vi "ListBox Auto Resize.vi"(8 "error in (no error)":errorcluster, 9 "Number of Columns":i32=4, 10 "Owning Pane":refnum<vi>, 11 "MultiColumn Listbox":refnum<vi>) -> (0 "error out":errorcluster)   [LabVIEW 2023]
uses:
  <vilib>/Utility/miscctls.llb/LVRowAndColumnTypeDef.ctl
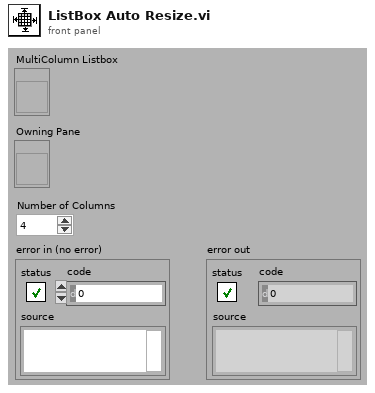
[diagram p1: front panel]
types:
  T1 = typedef "LVRowAndColumnTypeDef.ctl" = cluster{"Row":i32, "Column":i32}
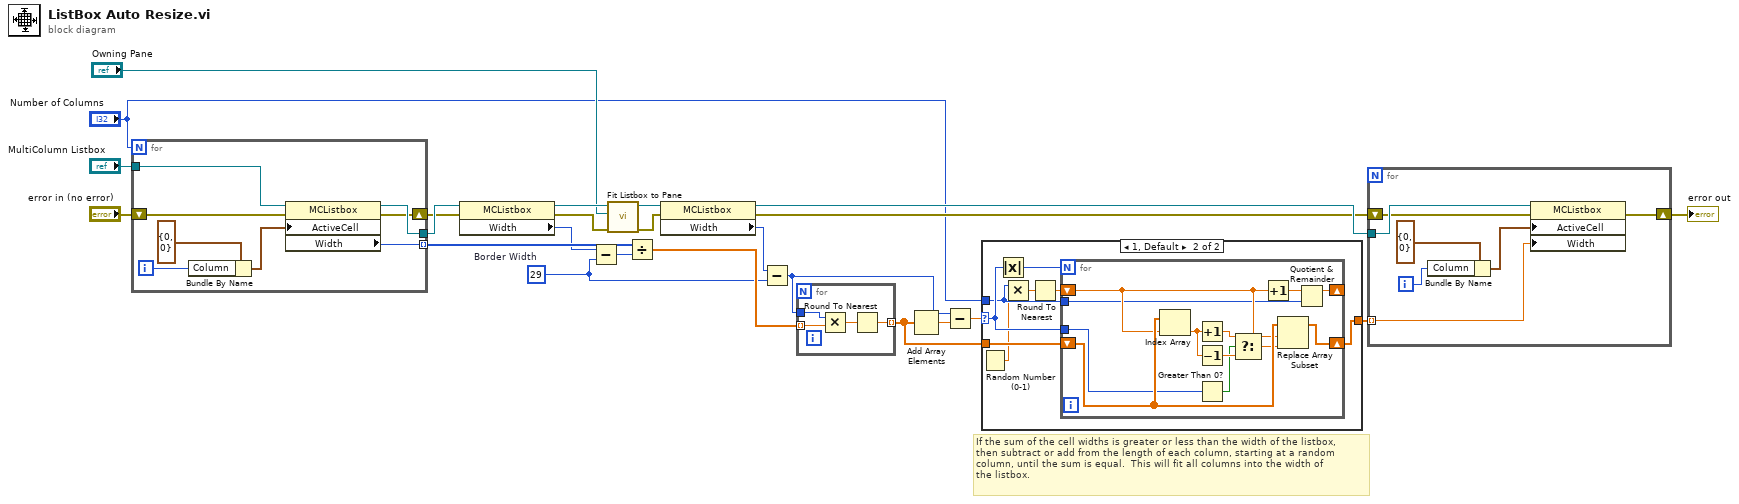
[diagram p0: block diagram]
diagram:
  w2 = u32 29  # Border Width
  # "If the sum of the cell widths is greater or less than the width of the listbox,\nthen subtract or add from the length of each column, starting at a random\ncolumn, until the sum is equal.  This will fit all columns into the width of \nthe listbox."
  n1 = for {
    N: "Number of Columns" -> [_]
    tunnel: "MultiColumn Listbox" -> [w32]
    tunnel: [w28] -> w6 mode=indexing
    tunnel: [w27] -> w24
    shift-right: [w25] -> w20
    shift-left: "error in (no error)" -> [w26]
    i -> [w30]
    n2 = Bundle By Name(cluster=T1 {"Row"=0, "Column"=0} ("Active Cell:Active Cell"), "Column"=w30) -> (w29:T1)
    n3 = property class="MCListbox"(reference=w32, error in=w26, "ActiveCell"=w29) -> (reference out=w27:refnum<vi>, error out=w25:errorcluster, "Width"=w28:u32)
  }
  n4 = property class="MCListbox"(reference=w24, error in=w20) -> (reference out=w14:refnum<vi>, error out=w15:errorcluster, "Width"=w5:u32)
  n5 = Subtract(x=w5, y=w2) -> (x-y=w4:u32)
  n6 = call "Fit Listbox to Pane.vi"("error in (no error)"=w15, "Owning Pane"="Owning Pane", "Multicolumn Listbox"=w14) -> ("error out"=w17:errorcluster, "Multicolumn Listbox"=w16:refnum<vi>)  [unwired: 7 in]
  n7 = Divide(x=w6, y=w4) -> (x/y=w12:dbl[])
  n8 = property class="MCListbox"(reference=w16, error in=w17) -> (reference out=w23:refnum<vi>, error out=w19:errorcluster, "Width"=w3:u32)
  n9 = Subtract(x=w3, y=w2) -> (x-y=w1:u32)
  n10 = for {
    tunnel: w12 -> [w36] mode=indexing
    tunnel: w1 -> [w35]
    tunnel: [w33] -> w8 mode=indexing
    n11 = Multiply(x=w35, y=w36) -> (x*y=w34:dbl)
    n12 = Round To Nearest(number=w34) -> (nearest integer value=w33:dbl)
  }
  n13 = Add Array Elements(numeric array=w8) -> (sum=w11:dbl)
  n14 = Subtract(x=w1, y=w11) -> (x-y=w10:dbl)
  n15 = case shown="1, Default" w10 {
    selector: w10 -> [_ w43]
    tunnel: "Number of Columns" -> [_ w41]
    tunnel: w8 -> [w37 w45]
    tunnel: [w37 w44] -> w7
    frame 0 {
    }
    frame 1, Default {
      n16 = Random Number (0-1)() -> (number: 0 to 1=w40:dbl)
      n17 = Absolute Value(x=w43) -> (abs(x)=w42:i32)
      n18 = Multiply(x=w41, y=w40) -> (x*y=w39:dbl)
      n19 = Round To Nearest(number=w39) -> (nearest integer value=w38:dbl)
      n20 = for {
        N: w42 -> [_]
        tunnel: w41 -> [w47]
        tunnel: w43 -> [w55]
        shift-right: [w56] -> w44
        shift-left: w45 -> [w57]
        shift-right: [w46] -> _
        shift-left: w38 -> [w49]
        n21 = Index Array(array=w57, index=w49) -> (element=w54:dbl)
        n22 = Increment(x=w54) -> (x+1=w53:dbl)
        n23 = Decrement(x=w54) -> (x-1=w52:dbl)
        n24 = Greater Than 0?(x=w55) -> (x > 0?=w50:bool)
        n25 = Select(t=w53, s=w50, f=w52) -> (s? t:f=w51:dbl)
        n26 = Increment(x=w49) -> (x+1=w48:dbl)
        n27 = Replace Array Subset(array=w57, new element=w51, index=w49) -> (w56:dbl[])
        n28 = Quotient & Remainder(x=w48, y=w47) -> (x-y*floor(x/y)=w46:dbl)  [unwired: 1 out]
      }
    }
  }
  n29 = for {
    tunnel: w23 -> [w61]
    shift-right: [w59] -> w18
    shift-left: w19 -> [w60]
    tunnel: w7 -> [w58] mode=indexing
    i -> [w62]
    n30 = Bundle By Name(cluster=T1 {"Row"=0, "Column"=0} ("Active Cell:Active Cell"), "Column"=w62) -> (w64:T1)
    n31 = property class="MCListbox"(reference=w61, error in=w60, "ActiveCell"=w64, "Width"=w58) -> (error out=w59:errorcluster)  [unwired: 1 out]
  }
  "error out" <- w18
